vi "rename channel.vi"(8 "error in":errorcluster, 9 "new channel name":string, 10 "old channel name":string, 11 "Scan Engine editor node in":refnum<class "Scan Engine editor node.lvclass">) -> (0 "error out":errorcluster, 3 "Scan Engine editor node out":refnum<class "Scan Engine editor node.lvclass">)   [LabVIEW 2013, in "Scan Engine editor node.lvclass"]
uses:
  Scan Engine editor node.lvclass
  read actual configuration.vi
  write actual configuration.vi
  <vilib>/NI/TBM Modules/variable/module/configuration/Scan Engine configuration.lvclass
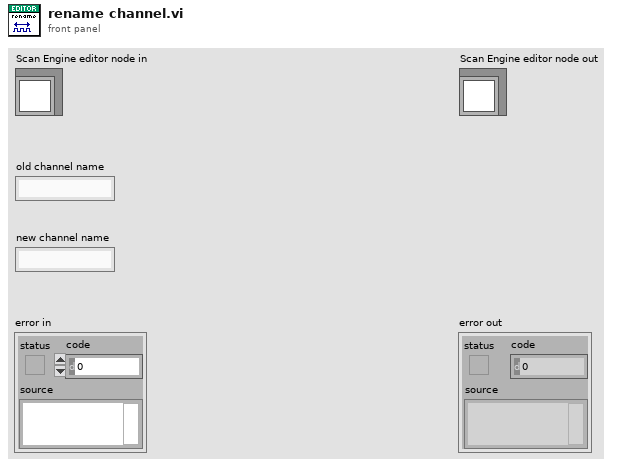
[diagram p1: front panel]
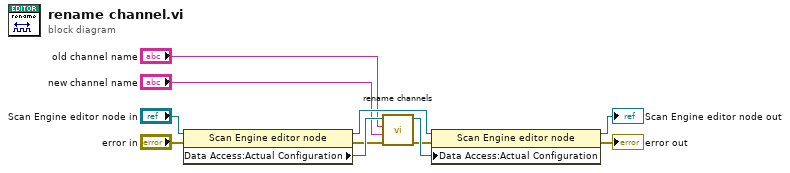
[diagram p0: block diagram]
diagram:
  n1 = property class="Scan Engine editor node"(reference="Scan Engine editor node in", error in="error in") -> (reference out=w8:refnum<class "Scan Engine editor node.lvclass">, error out=w1:errorcluster, "Data Access:Actual Configuration"=w6:refnum<class "Scan Engine configuration.lvclass">)
  n2 = call <vilib>:"rename channels.vi"("error in"=w1, "new name"="new channel name", "old name"="old channel name", "Scan Engine configuration in"=w6) -> ("error out"=w4:errorcluster, "Scan Engine configuration out"=w5:refnum<class "Scan Engine configuration.lvclass">)  [unwired: 6 in]
  n3 = property class="Scan Engine editor node"(reference=w8, error in=w4, "Data Access:Actual Configuration"=w5) -> (reference out=→"Scan Engine editor node out":refnum<class "Scan Engine editor node.lvclass">, error out=→"error out":errorcluster)
